vi "SSL Detection Frame Balls Kalman Estimator.vi"(5 "Time Stamp 2":timestamp=timestamp(3583818425.330139 s since 1904-01-01), 7 "Life Time 2":dbl=0.2, 11 "Detection Ball \nArray":T1[](array[typedef])) -> (3 "balls":T1[](array[typedef]))   [LabVIEW 2023]
uses:
  Controls/SSL Detection Ball.ctl
  <vilib>/Analysis/Matrix/Datatypes/RealMatrix.ctl
  <vilib>/Analysis/_algsub.llb/Real Vector Norm.vi
  <vilib>/Analysis/Matrix/Numeric/Subtract/Subtract - RM,RM.vi
  <vilib>/Analysis/Matrix/NI_Matrix.lvlib
  <vilib>/Analysis/NI_AALPro.lvlib
panel:
  in  "Life Time":dbl=2.0
  in  "Array":T3(array[cluster])
  out "A - B":dbl[][](array[numeric])
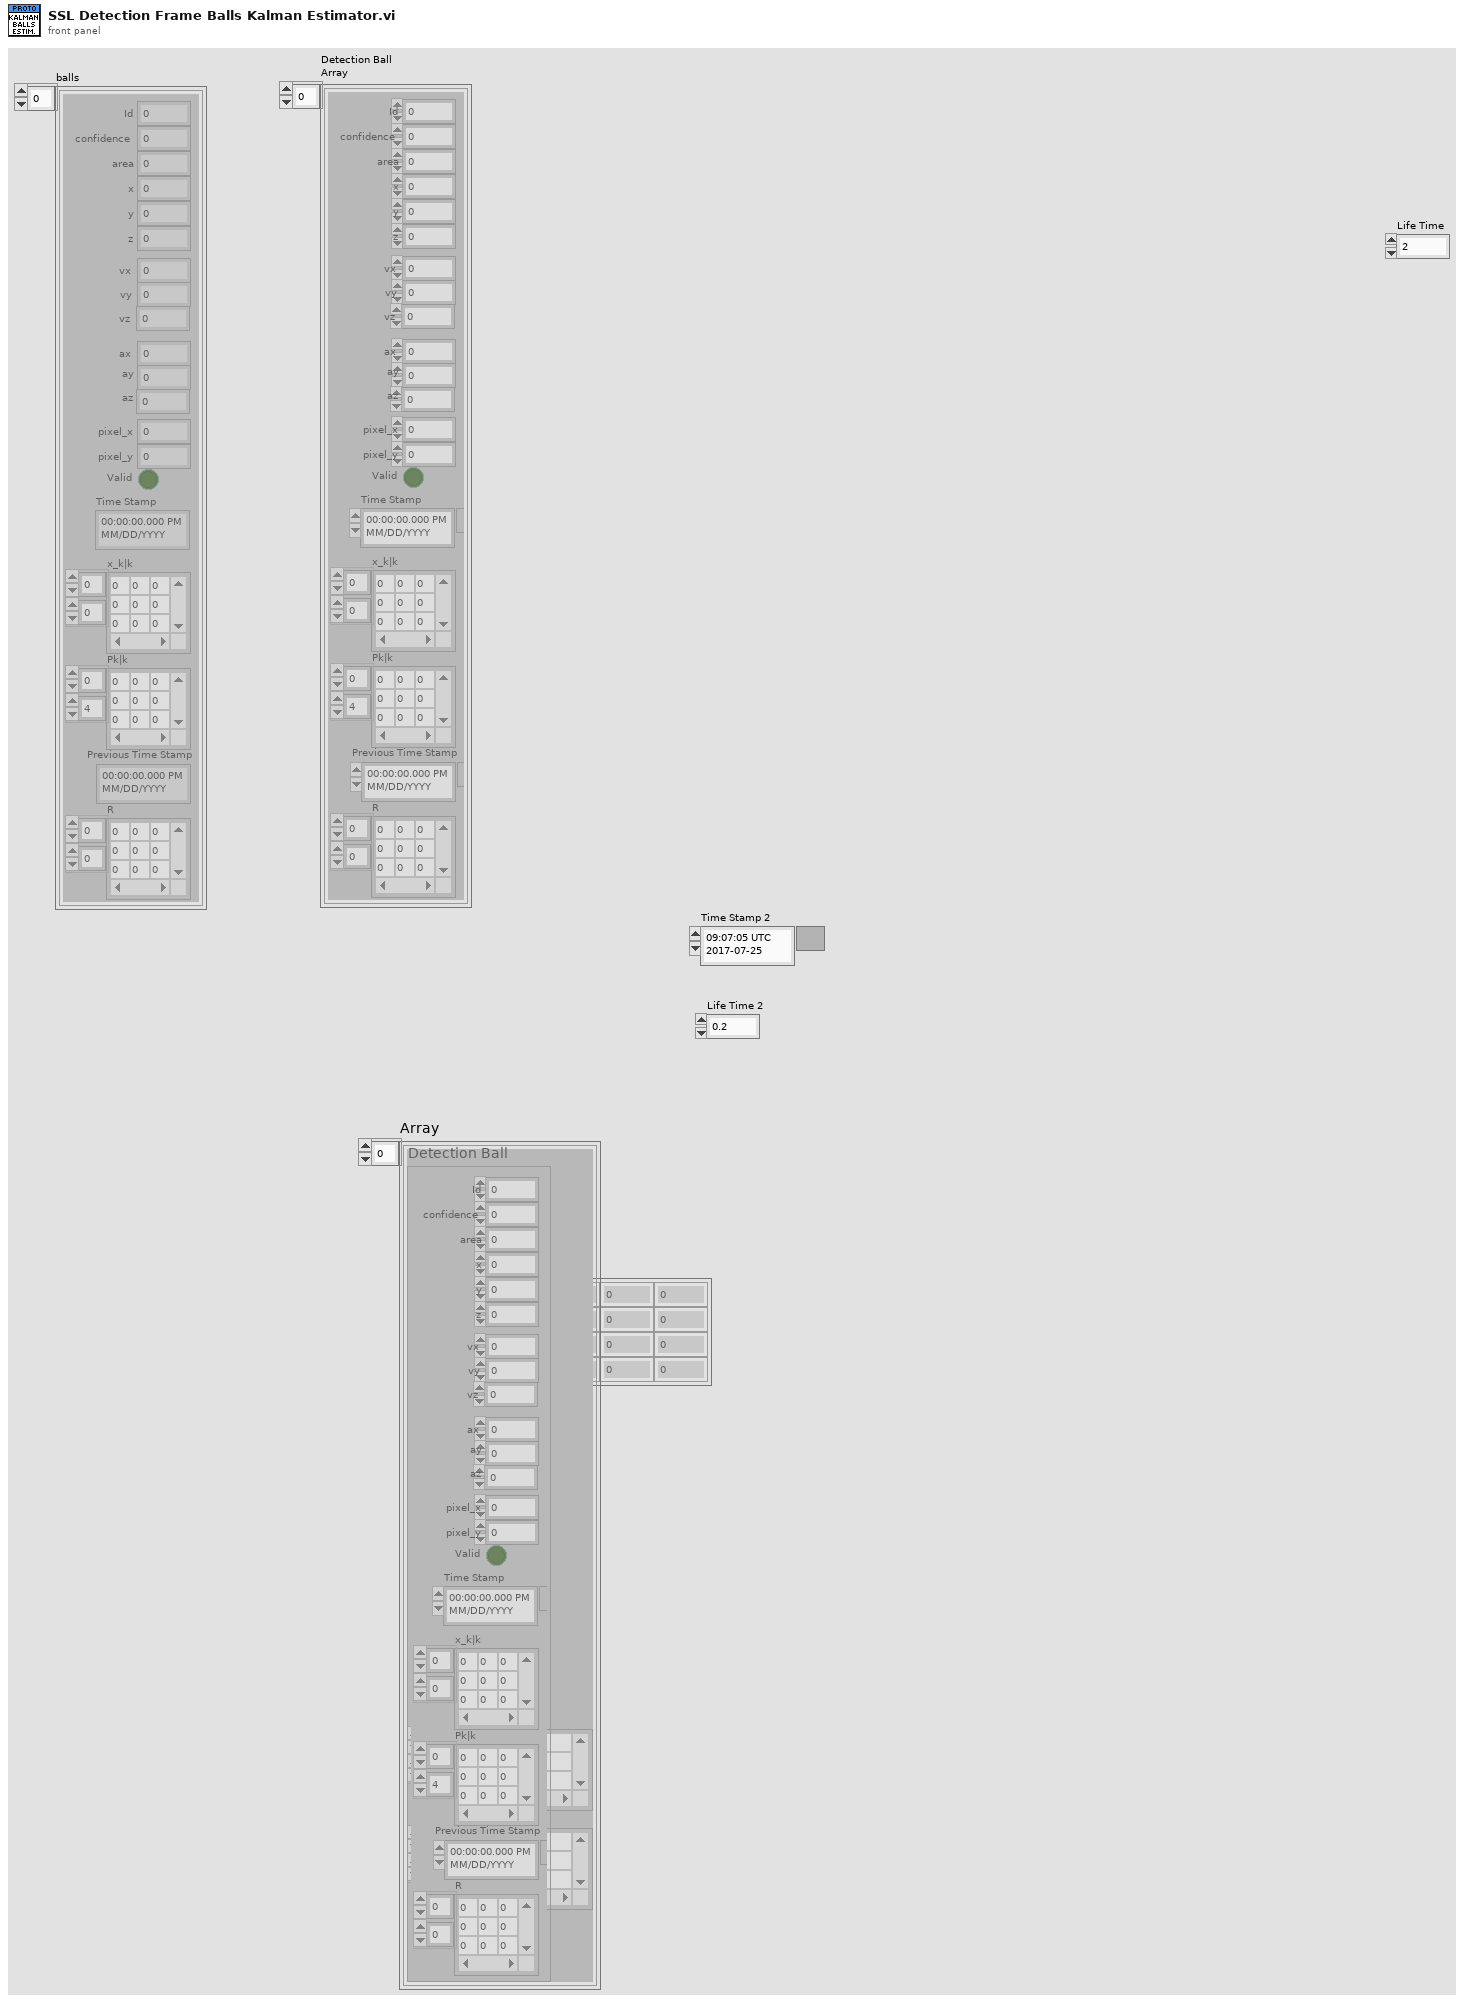
[diagram p1: front panel]
types:
  T1 = typedef "SSL Detection Ball.ctl" = cluster{"x":sgl, "area":u32, "confidence":sgl, "y":sgl, "z":sgl, "pixel_x":sgl, "pixel_y":sgl, "Valid":bool, "Time Stamp":timestamp, "x_k|k":T2, "Pk|k":T2, "Id":u32, "Previous Time Stamp":timestamp, "R":T2, " vx":sgl, "vy":dbl, "vz":dbl, " ax":sgl, "ay":dbl, "az":dbl}
  T2 = typedef "NI_Matrix.lvlib/RealMatrix.ctl" = dbl[][]
  T3 = cluster{"Detection Ball":T1, "Pose":T2, "Pk|k":T2}[]
  T4 = cluster{"Detection Ball":T1, "Pose":T2, "Pk|k":T2}
  T5 = cluster{"Detection Ball out":T1, "x_k|k":T2, "Pk|k":T2}
  T6 = typedef "SSL Detection Ball.ctl" = cluster{"x":sgl, "area":u32, "confidence":sgl, "y":sgl, "z":sgl, "pixel_x":sgl, "pixel_y":sgl, "Valid":bool, "Time Stamp":timestamp, "x_k|k":T2, "Pk|k":T2, "ID#":dbl}
  T7 = cluster{"Detection Ball out":T1, "x_k|k":T2, "Pk|k":T2}[]
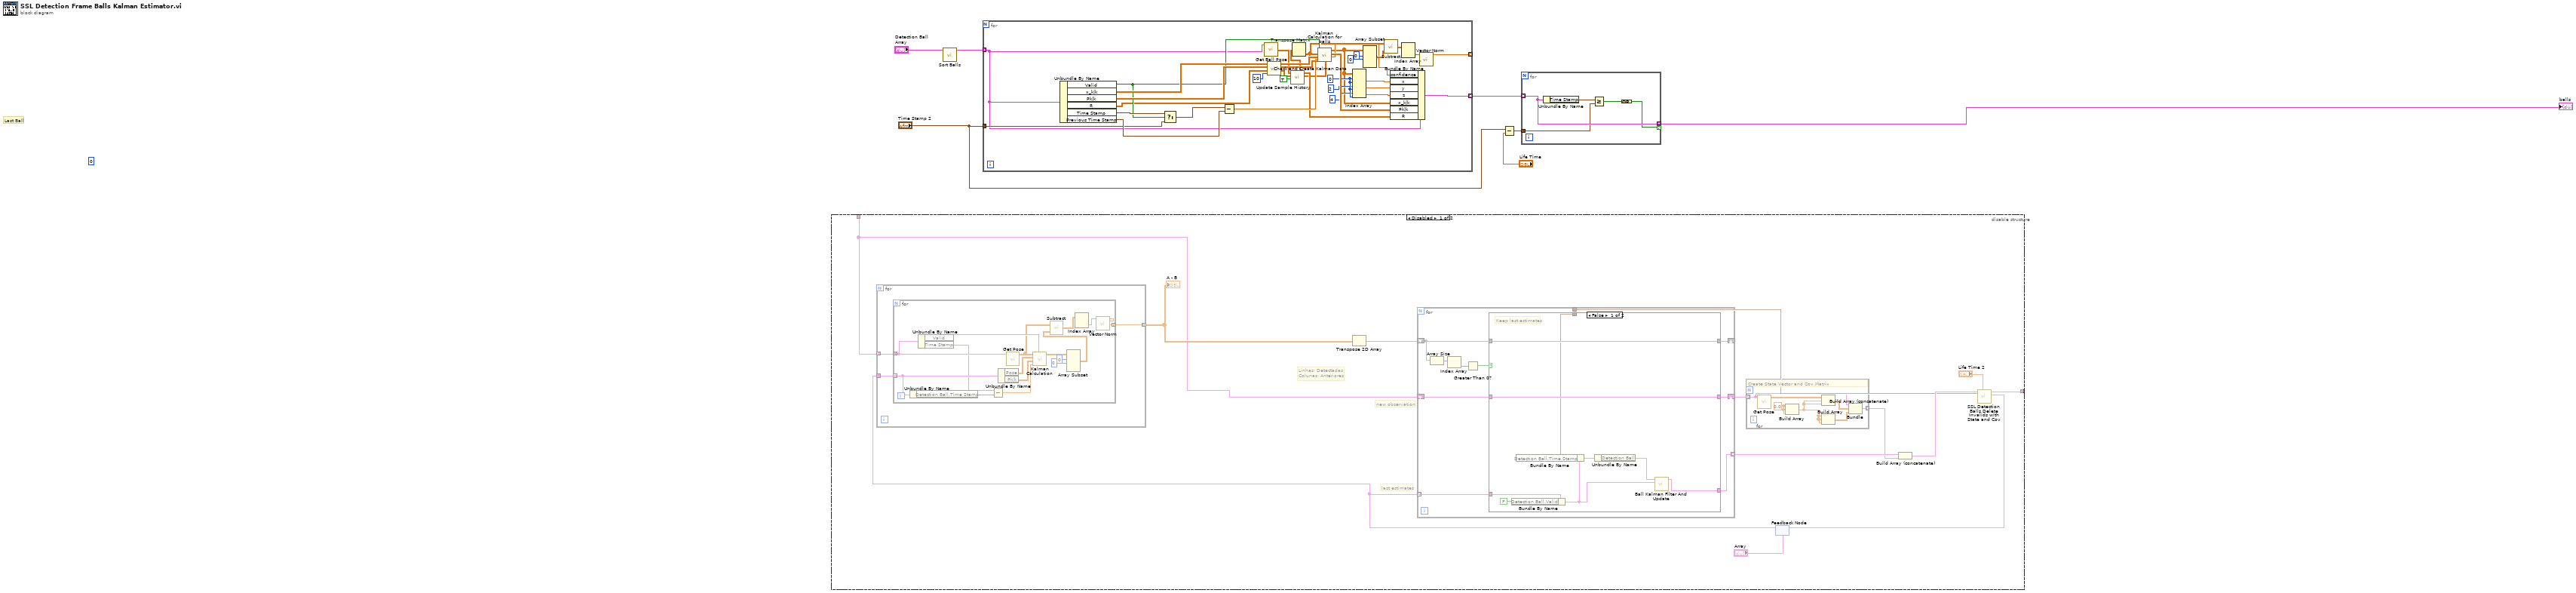
[diagram p0: block diagram]
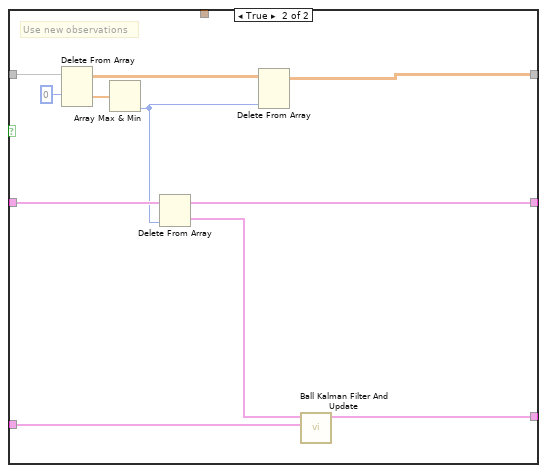
[diagram p2: hidden frame]
diagram:
  (unwired) u32 0 ("ID#")
  # "Last Ball"
  n1 = disable-structure shown="Disabled" {
    disable-tunnel: _ -> [w17 _]
    disable-tunnel: [w9 _] -> _
    frame Disabled {
      # "last estimates"
      # "new observation"
      # "Linhas: Detectadas\nColunas: Anteriores"
      n2 = feedback #1("Array") -> (w11:T3)
      n3 = for {
        tunnel: w11 -> [w60]
        tunnel: w17 -> [w59] mode=indexing
        tunnel: [w58] -> w19 mode=indexing
        n4 = for {
          tunnel: w60 -> [w64] mode=indexing
          tunnel: w59 -> [w76]
          tunnel: [w69] -> w58 mode=indexing
          n5 = Unbundle By Name(w64) -> ("Detection Ball.Time Stamp"=w63:timestamp)
          n6 = Unbundle By Name(w76) -> ("Valid"=w75, "Time Stamp"=w62)
          n7 = Subtract(x=w62, y=w63) -> (x-y=w61:dbl)
          n8 = Unbundle By Name(w64) -> ("Pose"=w66:T2, "Pk|k"=w65:T2)
          n9 = call-poly "Get Pose.vi"("Detection Ball"=w76) -> ("Pose"=w74:T2)  [unwired: 10 in]
          n10 = call "Kalman Calculation.vi"("Use Observation"=w75, "intervalo"=w61, "Pk-1|k-1"=w65, "x_k-1|k-1"=w66, "z_k"=w74) -> ("x_k|k"=w72:T2)  [unwired: 4 in, 2 out]
          n11 = Array Subset(array=w72, index (row)=0 ("row 1"), length (row)=0 ("row N")) -> (w73:T2)  [unwired: 2 in]
          n12 = call-poly <vilib>:"Subtract.vi"("Real Matrix B"=w73, "Real Matrix A"=w74) -> ("A - B"=w68:T2)
          n13 = Index Array(array=w68) -> (element=w67:dbl[])  [unwired: 2 in]
          n14 = call-poly <vilib>:"Vector Norm.vi"("Input Vector"=w67) -> ("norm"=w69:dbl)  [unwired: 9 in, 1 out]
        }
      }
      "A - B" <- w19
      n15 = Transpose 2D Array(2D array=w19) -> (transposed array=w20:dbl[][])
      n16 = for {
        shift-right: [w36] -> _
        shift-left: w20 -> [w32]
        shift-right: [w35] -> w18
        shift-left: w17 -> [w37]
        tunnel: [w34] -> w16 mode=indexing
        tunnel: w11 -> [w33] mode=indexing
        tunnel: w10 -> [w28]
        n17 = Array Size(array=w32) -> (size(s)=w30:i32[])
        n18 = Index Array(array=w30) -> (element=w29:i32)  [unwired: 1 in]
        n19 = Greater Than 0?(x=w29) -> (x > 0?=w31:bool)
        n20 = case shown="False" w31 {
          tunnel: w32 -> [w46 w57]
          tunnel: w37 -> [w45 w54]
          tunnel: [w46 w52] -> w36
          tunnel: [w45 w50] -> w35
          tunnel: [w38 w49] -> w34
          tunnel: w33 -> [w43 w47]
          tunnel: w28 -> [w41 _]
          frame False {
            # "Keep last estimates"
            n21 = Bundle By Name(cluster=w43, "Detection Ball.Valid"=FALSE) -> (w42:T4)
            n22 = Bundle By Name(cluster=w42, "Detection Ball.Time Stamp"=w41) -> (w40:T4)
            n23 = Unbundle By Name(w40) -> ("Detection Ball"=w39:T1)
            n24 = call "Ball Kalman Filter And Update.vi"("Cluster in"=w42, "Detection Ball"=w39) -> ("Cluster out"=w38:T5)  [unwired: 9 in]
          }
          frame True {
            # "Use new observations"
            n25 = Delete From Array(array=w57, index (row)=0) -> (deleted portion=w55:dbl[], array with subset deleted=w53:dbl[][])  [unwired: 2 in]
            n26 = Array Max & Min(array=w55) -> (min index (indices)=w51:i32)  [unwired: 3 out]
            n27 = Delete From Array(array=w54, index=w51) -> (deleted portion=w48:T6, array with subset deleted=w50:T6[])  [unwired: 1 in]
            n28 = Delete From Array(array=w53, index (col)=w51) -> (array with subset deleted=w52:dbl[][])  [unwired: 2 in, 1 out]
            n29 = call "Ball Kalman Filter And Update.vi"("Cluster in"=w47, "Detection Ball"=w48) -> ("Cluster out"=w49:T5)  [unwired: 9 in]
          }
        }
      }
      n30 = for {
        tunnel: w18 -> [w21] mode=indexing
        tunnel: [w22] -> w15 mode=indexing
        w27 = 0.0 ("element")
        # "Create State Vector and Cov Matrix"
        n31 = call-poly "Get Pose.vi"("Detection Ball"=w21) -> ("Pose"=w25:T2)  [unwired: 10 in]
        n32 = Build Array(w27, w27, w27) -> (w26:dbl[])
        n33 = Build Array(w26, w26, w26) -> (w24:dbl[][])
        n34 = Build Array (concatenate)(w25, w26, w26) -> (w23:T2)
        n35 = Bundle("Detection Ball"=w21, "Pose"=w23, w24) -> (w22:cluster{"Detection Ball":T6, "Pose":T2, dbl[][]})  [unwired: 1 in]
      }
      n36 = Build Array (concatenate)(w16, w15) -> (w13:T7)
      n37 = call "SSL Detection Balls Delete Invalids with State and Cov.vi"("Life Time"="Life Time 2", "Array"=w13) -> ("Array 2"=w8:T3, "Balls Out"=w9:T1[], "Now"=w10:timestamp)  [unwired: 7 in]
      n38 = feedback-in #1(w8) -> ()
    }
    frame Enabled {
    }
  }
  n39 = call "Sort Balls.vi"("Detection Ball \nArray"="Detection Ball \nArray") -> ("Sorted Detection Ball \nArray"=w3:T1[])  [unwired: 10 in]
  n40 = for {
    tunnel: w3 -> [w78] mode=indexing
    tunnel: [w112] -> _ mode=indexing
    tunnel: [w82] -> w5 mode=indexing
    tunnel: "Time Stamp 2" -> [w98]
    w93 = 0 ("index (row)")
    n41 = Unbundle By Name(w78) -> ("Valid"=w96:bool, "x_k|k"=w105:T2, "Pk|k"=w103:T2, "R"=w90:T2, "Time Stamp"=w99:timestamp, "Previous Time Stamp"=w101:timestamp)
    n42 = Select(t=w99, s=w96, f=w98) -> (s? t:f=w97:timestamp)
    n43 = Subtract(x=w97, y=w101) -> (x-y=w100:dbl)
    n44 = call "Get Ball Pose.vi"("Detection Ball"=w78) -> ("Pose"=w81:T2)  [unwired: 10 in]
    n45 = call "Check and Create Kalman Data.vi"("Variance Memory"=10, "R"=w90, "Pk"=w103, "x_k"=w105) -> ("R out"=w89:T2, "Pk out"=w102:T2, "x_k out"=w104:T2)  [unwired: 5 in]
    n46 = call "Update Sample History.vi"("Ball?"=TRUE, "R in"=w89, "Sample"=w81) -> ("covariance matrix V"=w85:T2, "R out"=w86:T2, "Sample Unwrapped"=w84:T2)  [unwired: 6 in]
    n47 = Transpose Matrix(1:w84) -> (0:w87:T2)
    n48 = call "Kalman Calculation for balls.vi"("R"=w85, "intervalo"=w100, "Pk-1|k-1"=w102, "x_k-1|k-1"=w104, "z_k"=w87, "Use Observation"=w96) -> ("Conf"=w83:dbl, "Pk|k"=w106:T2, "x_k|k"=w80:T2)  [unwired: 3 in]
    n49 = Index Array(array=w80, index (row) #1=w93, index (col) #1=w93, index (row) #2=2 ("disabled index (col)"), index (col) #2=w93, index (row) #3=4 ("disabled index (col)"), index (col) #3=w93) -> (element #1=w95:dbl, element #2=w94:dbl, element #3=w77:dbl)
    n50 = Array Subset(array=w80, index (row)=0 ("row 1"), length (row)=0 ("row N")) -> (w111:T2)  [unwired: 2 in]
    n51 = call-poly <vilib>:"Subtract.vi"("Real Matrix B"=w111, "Real Matrix A"=w87) -> ("A - B"=w108:T2)
    n52 = Bundle By Name(cluster=w78, "confidence"=w83, "x"=w95, "y"=w94, "z"=w77, "x_k|k"=w80, "Pk|k"=w106, "R"=w86) -> (w82:T1)
    n53 = Index Array(array=w108) -> (element=w107:dbl[])  [unwired: 2 in]
    n54 = call-poly <vilib>:"Vector Norm.vi"("Input Vector"=w107) -> ("norm"=w112:dbl)  [unwired: 9 in, 1 out]
  }
  n55 = Subtract(x="Time Stamp 2", y="Life Time") -> (x-y=w6:timestamp)
  n56 = for {
    tunnel: w5 -> [w117] mode=indexing
    tunnel: [w117] -> w1 mode=indexing if=w116
    tunnel: w6 -> [w114]
    n57 = Unbundle By Name(w117) -> ("Time Stamp"=w115:timestamp)
    n58 = Greater Or Equal?(x=w115, y=w114) -> (x >= y?=w113:bool)
    n59 = Compound Arithmetic op=OR(w113) -> (w116:bool)
  }
  "balls" <- w1
